vi "MAIN_move_to_XY_positions.vi"(7 "queue ASI stage":refnum<queue>, 8 "error out":errorcluster, 9 "ROI manager":i32(listbox), 10 "ROI manager":refnum<vi>, 11 "XY positions":dbl[][](array[numeric])) -> (0 "error out":errorcluster, 2 "Next task":T1, 3 "ROI manager out":i32, 5 "XY positions":dbl[][](array[numeric]))   [LabVIEW 2015]
uses:
  CONTROLS/Q_ASI_stage_element.ctl
  CONTROLS/Q_main_element.ctl
panel:
  in  "Start acquisition":bool
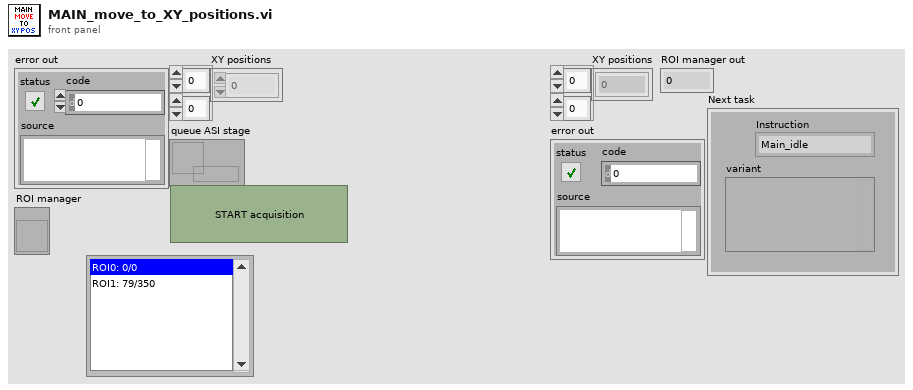
[diagram p1: front panel]
types:
  T1 = typedef "Q_main_element.ctl" = cluster{"variant":variant, "Instruction":enum16{"Main_idle", "Main_initialize", "Main_initialize_TDMS", "Main_initialize_Queue", "Main_error", "Main_DAQ_initialization_results", "Main_ASI_initialization_results", "Main_Piezo_initialization_results", "Main_Valve_initialization_results", "Main_Pump_initialization_results", "Main_CAMERA_initialization_results", "Main_FPGA_initialization_results", "Main_DAQ_error", "Main_ASI_error", "Main_Piezo_error", "Main_CAMERA_error", "Main_Valve_error", "Main_Pump_error", "Main_FPGA_error", "Main_start_acquiring", "Main_not_acquiring", "Main_acquiring", "Main_stop_acquiring", "Main_change_exposure", "Main_change_z_scan_parameters", "Main_define_ROI", "Main_define_mosaic", "Main_read_kinetic_time", "Main_cooler", "Main_read_temperature", "Main_save_XY", "Main_load_XY", "Main_discard_XY", "Main_move_to_XY", "Main_measure_QPD", "Main_autofocus_calibration", "Main_autofocus_initialization", "Main_autofocus_stop", "Main_save_PID", "Main_change_H_valve_position", "Main_two_way_valve", "Main_save_movie", "Main_init_single_scan", "Main_single_scan", "Main_stop_single_scan", "Main_merFISH_illumination_parameters", "Main_merFISH_buffer_probe_list", "Main_merFISH_injections_procedure", "Main_merFISH_save_setpoint", "Main_merFISH_DAPI_parameters", "Main_merFISH_Brightfield_parameters", "Main_merFISH_save_embryo_ROI", "Main_merFISH_init", "Main_merFISH_resume", "Main_merFISH_start_autofocus", "Main_merFISH_open_close_valve_merFISH", "Main_merFISH_open_close_valve_photobleaching", "Main_merFISH_hybridization", "Main_merFISH_move_to_ROI", "Main_merFISH_wait_stabilization", "Main_merFISH_move_to_REF", "Main_merFISH_scan", "Main_merFISH_photobleaching_injection", "Main_merFISH_photobleaching", "Main_merFISH_send_email", "Main_merFISH_close", "Main_STOP"}}
  T2 = enum16{"Left Button", "Center Button", "Right Button", "Window Close"}
  T3 = typedef "Q_ASI_stage_element.ctl" = cluster{"variant":variant, "Instruction":enum16{"ASI_idle", "ASI_initialize", "ASI_error", "ASI_security_stop", "ASI_read_XYZ", "ASI_up", "ASI_down", "ASI_left", "ASI_right", "ASI_save_XY", "ASI_move_to_XY", "ASI_brightfield", "ASI_init_scan", "ASI_init_merFISH", "ASI_move_to_XY_merFISH", "ASI_move_to_Z_merFISH", "ASI_init_autofocus_search_merFISH", "ASI_close_autofocus_search_merFISH", "ASI_adjust_piezo_autofocus_merFISH", "ASI_set_piezo_autofocus_to_reference_position_merFISH_TL", "ASI_close_merFISH", "ASI_stop"}}
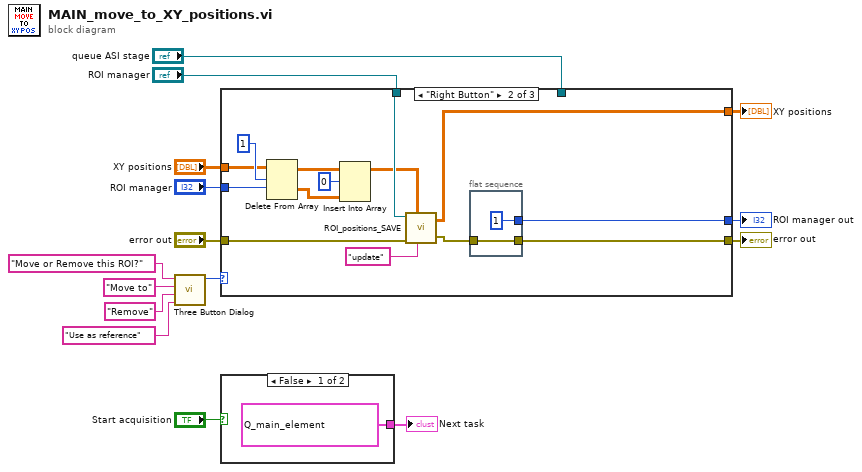
[diagram p0: block diagram]
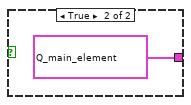
[diagram p2: hidden frame]
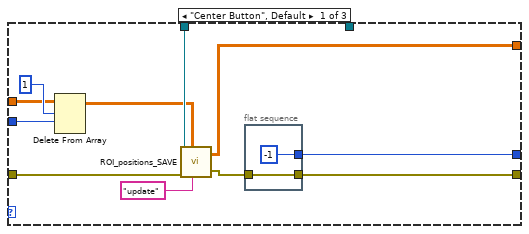
[diagram p3: hidden frame]
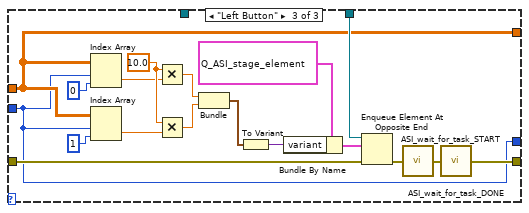
[diagram p4: hidden frame]
diagram:
  n1 = call <vilib>:"Three Button Dialog.vi"("Right Button Text (\"Cancel\")"="Use as reference" ("Right Button Text (\"Cancel\")"), "Center Button Text (\"No\")"="Remove" ("F button name (\"Cancel\")"), "Left Button Text (\"Yes\")"="Move to" ("T button name (\"OK\")"), "message"="Move or Remove this ROI?") -> ("Which Button?"=w15:T2)  [unwired: 7 in]
  n2 = case shown="\"Right Button\"" w15 {
    tunnel: "ROI manager" -> [w25 w41 w45]
    tunnel: "queue ASI stage" -> [_ _ w51]
    tunnel: "error out" -> [w18 w35 w50]
    tunnel: [w21 w37 w47] -> w3
    tunnel: "ROI manager" -> [w20 w36 _]
    tunnel: [w23 w39 w46] -> w4
    tunnel: "XY positions" -> [w17 w30 w46]
    tunnel: [w16 w29 w45] -> w2
    frame "Center Button", Default {
      n3 = Delete From Array(array=w17, length=1, index (row)=w25) -> (array with subset deleted=w19:dbl[][])  [unwired: 1 in, 1 out]
      n4 = call "ROI_positions_SAVE.vi"("Choice"="update", "XY positions"=w19, "error in"=w18, "ROI LstBox Refnum"=w20) -> ("error out"=w22:errorcluster, "XY positions OUT"=w23:dbl[][])  [unwired: 2 in]
      n5 = flat-sequence {
        tunnel: w22 -> [w28]
        tunnel: [w28] -> w21
        tunnel: [-1 ("ROI manager")] -> w16
        frame #0 {
        }
      }
    }
    frame "Right Button" {
      n6 = Delete From Array(array=w30, length=1, index (row)=w41) -> (deleted portion=w32:dbl[][], array with subset deleted=w34:dbl[][])  [unwired: 1 in]
      n7 = Insert Into Array(array=w34, index (row)=0, new element=w32) -> (w31:dbl[][])  [unwired: 1 in]
      n8 = call "ROI_positions_SAVE.vi"("Choice"="update", "XY positions"=w31, "error in"=w35, "ROI LstBox Refnum"=w36) -> ("error out"=w38:errorcluster, "XY positions OUT"=w39:dbl[][])  [unwired: 2 in]
      n9 = flat-sequence {
        tunnel: w38 -> [w44]
        tunnel: [w44] -> w37
        tunnel: [1 ("ROI manager")] -> w29
        frame #0 {
        }
      }
    }
    frame "Left Button" {
      w60 = 10.0
      n10 = Index Array(array=w46, index (row)=w45, index (col)=0 ("disabled index (col)")) -> (element=w59:dbl)
      n11 = Index Array(array=w46, index (row)=w45, index (col)=1 ("disabled index (col)")) -> (element=w58:dbl)
      n12 = Multiply(x=w60, y=w59) -> (x*y=w57:dbl)
      n13 = Multiply(x=w60, y=w58) -> (x*y=w56:dbl)
      n14 = Bundle(w57, w56) -> (w55:cluster{dbl, dbl})  [unwired: 1 in]
      n15 = To Variant(anything=w55) -> (Variant=w53:variant)
      n16 = Bundle By Name(cluster=T3 {"variant"=variant, "Instruction"=enum."ASI_move_to_XY"} ("Q_ASI_stage"), "variant"=w53) -> (w52:T3)
      n17 = Enqueue Element At Opposite End(queue=w51, element=w52, error in (no error)=w50) -> (error out=w49:errorcluster)  [unwired: 1 in, 2 out]
      n18 = call "ASI_wait_for_task_START.vi"("error in"=w49) -> ("error out"=w48:errorcluster)
      n19 = call "ASI_wait_for_task_DONE.vi"("error in"=w48) -> ("error out"=w47:errorcluster)
    }
  }
  "XY positions" <- w4
  "error out" <- w3
  "ROI manager out" <- w2
  n20 = case shown="False" "Start acquisition" {
    tunnel: [T1 {"variant"=variant, "Instruction"=enum."Main_not_acquiring"} ("Q_main_element") T1 {"variant"=variant, "Instruction"=enum."Main_acquiring"} ("Q_main_element")] -> w1
    frame False {
    }
    frame True {
    }
  }
  "Next task" <- w1
